vi "TTA_MATLAB_TX_Perform1RFIC1TxACPRTest.vi"(0 "Channel":string(combo), 1 "MXG VISA Resource In":refnum<visa-resource-name>, 2 "EXA VISA Resource":refnum<visa-resource-name>, 5 "Tx":string(combo), 7 "Active ACPR Refnum":refnum<vi>, 11 "error in":errorcluster) -> (4 "ACPR\nResults":T1, 12 "MXG VISA Resource Out":refnum<visa-resource-name>, 13 "EXA VISA Resource Out":refnum<visa-resource-name>, 15 "error out":errorcluster)   [LabVIEW 2016]
uses:
  TTA_Globals/TTA_Global_Complete_Settings.vi
panel:
  out "RFPAL PMU\nResults":dbl[](array[numeric])
  out "RF Frequency":dbl[](array[numeric])
  out "ACPR Data":dbl[][](array[numeric])
  out "In Range?":bool[](array[boolean])
  out "Amp Max\nSpec (dBm)":dbl
  out "Amp Min\nSpec (dBm)":dbl
  out "IF Index":i32
  in  "PALLinearization Values":T2
  out "Tx#":i32
  out "CH#":i32
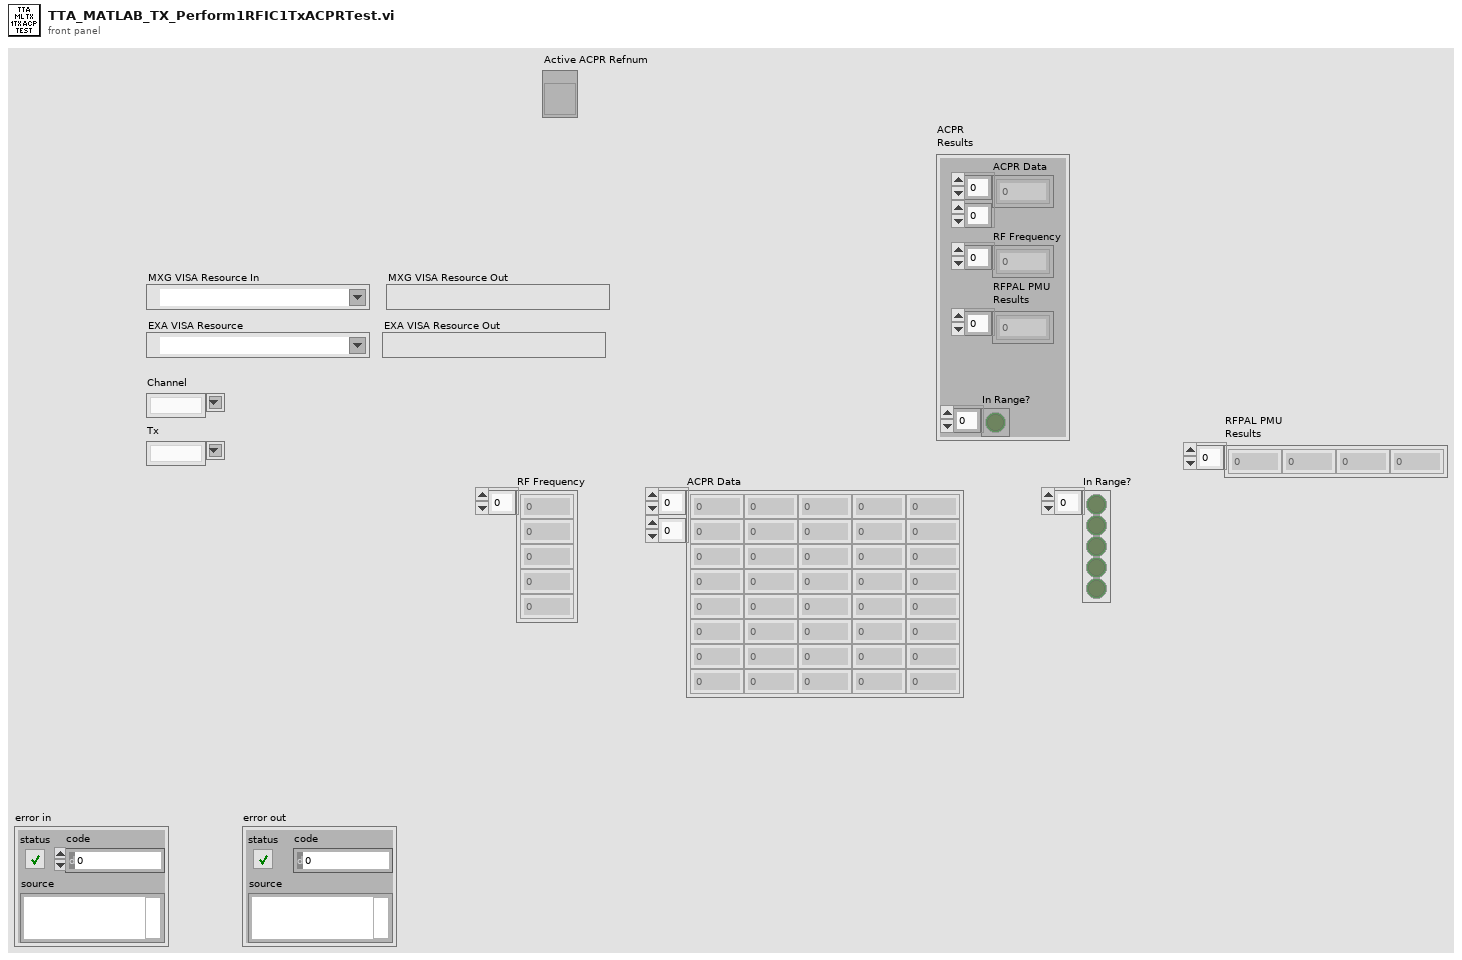
[diagram p1: front panel]
types:
  T1 = cluster{"ACPR Data":dbl[][], "RF Frequency":dbl[], "RFPAL PMU\nResults":dbl[], "In Range?":bool[]}
  T2 = cluster{"Tx IF Offsets":dbl[], "ACPR Filename":string, "Sampling Rate":dbl, "TxIF_Freq":dbl, "Power (dBm)":dbl, "IF Frequency Sweep (MHz)":dbl[], "BDSFreq":dbl, "Amplitude Range\nMax(dBm)":dbl, "Amplitude Range\nMin(dBm)":dbl, "CAL Amplitude\nIncrement(dB)":dbl, "CAL Amplitude\nDecrement (dB)":dbl, "Amplitude Least\nCriteria (dBm)":dbl}
  T3 = typedef "TTA_Control_Complete_Settings_Cluster.ctl" = cluster{"Brief Cluster":cluster{"STM Firmware File":string, "STM Firmware Address":string, "Required SW Version":string, "Template Used":string}, "Instrument Setting Cluster":cluster{"BDSFreq":dbl, "BDS Amp":dbl, "TxRFCal_Freq":dbl, "TxRFCal_Amp":dbl, "RxRFCal_Freq":dbl, "RxRFCal_Freq":dbl, "TxIF_Freq":dbl, "TxIF_Amp":dbl, "Tx_Output_Power_Signal_Freq":dbl, "Tx_ACPR_Signal_Freq":dbl, "Rx_RF_Freq":dbl, "Rx_RF_Amp":dbl, "Rx_Output_Power_Signal_Freq":dbl, "Rx_Output_Power_Sense_Freq":dbl}, "PAL Calibration\nInputs Cluster":cluster{"Amplitude Range\nMax(dBm)":dbl, "Amplitude Range\nMin(dBm)":dbl, "Amplitude Least\nCriteria (dBm)":dbl, "Frequency 1":dbl, "Frequency 2":dbl, "Frequency 3":dbl, "CAL Amplitude\nDecrement (dB)":dbl, "CAL Amplitude\nIncrement(dB)":dbl, "DownloadFile":string}, "TxOffset Cal Cluster":cluster{"Tx1 Offset (dB)":dbl, "Tx2 Offset (dB)":dbl, "Tx3 Offset (dB)":dbl, "Tx4 Offset (dB)":dbl, "Total RF Tx Loss (dB)":dbl}, "RxOffset Cal Cluster":cluster{"Rx1 Offset (dB)":dbl, "Rx2 Offset (dB)":dbl, "Rx3 Offset (dB)":dbl, "Rx4 Offset (dB)":dbl, "Total RF Rx Loss (dB)":dbl}, "TX Output Power Settings Cluster":cluster{"Frequency Sweep (MHz)":dbl[], "Sig Gen \nPower (dBm)":dbl, "Span (kHz)":dbl, "RBW (Hz)":dbl, "Ref Level (dBm)":dbl, "Low Power \nLimit":dbl, "High Power \nLimit":dbl, "DigAtt Max":dbl, "DigAtt Min":dbl}, "Tx ACPR Settings Cluster":cluster{"ACPR Filename":string, "Sampling Rate":dbl, "Power (dBm)":dbl, "IF Frequency Sweep (MHz)":dbl[], "State Name":string, "Mechanical\nAttenuation":dbl, "RefLevel Offset":dbl, "Amplitude Range\nMax (dBm)":dbl, "Amplitude Range\nMin (dBm)":dbl, "Cal Amp \nIncrement (dB)":dbl, "Cal Amp\nDecrement (dB)":dbl}, "Power Cal Cluster":cluster{"Power List (dBm)":dbl[], "Frequency (MHz)":dbl[], "Cal Decrement (dB)":dbl, "Cal Increment (dB)":dbl}, "Rx Received Power Settings Cluster":cluster{"Frequency Sweep (MHz)":dbl[], "Power (dBm)":dbl, "Span (kHz)":dbl, "RBW (Hz)":dbl, "Ref Level":dbl, "Low Power \nLimit (dBm)":dbl, "High Power\nLimit (dBm)":dbl}, "Tx Output Power Criteria Cluster":cluster{"CH1-TX1 \nMin":dbl, "CH1-TX1\nMax":dbl, "CH1-TXx3\nMin ":dbl, "CH1-TXx3\nMax":dbl, "CH2-TX1\nMin":dbl, "CH2-TX1\nMax":dbl, "CH2-TXx3\nMin":dbl, "CH2-TXx3\nMax":dbl}, "Tx ACPR Criteria Cluster":cluster{"Min Inband":dbl, "Max Close Outband":dbl, "Max Far Outband":dbl}, "Rx Output Power Criteria Cluster":cluster{"CH1-RX1 \nMin":dbl, "CH1-RX1 \nMax":dbl, "CH1-RXx3 \nMin":dbl, "CH1-RXx3\nMax":dbl, "CH2-RX1\nMin":dbl, "CH2-RX1\nMax":dbl, "CH2-RXx3\nMin":dbl, "CH2-RXx3\nMax":dbl}}
  T4 = cluster{"BDSFreq":dbl, "BDS Amp":dbl, "TxRFCal_Freq":dbl, "TxRFCal_Amp":dbl, "RxRFCal_Freq":dbl, "RxRFCal_Freq":dbl, "TxIF_Freq":dbl, "TxIF_Amp":dbl, "Tx_Output_Power_Signal_Freq":dbl, "Tx_ACPR_Signal_Freq":dbl, "Rx_RF_Freq":dbl, "Rx_RF_Amp":dbl, "Rx_Output_Power_Signal_Freq":dbl, "Rx_Output_Power_Sense_Freq":dbl}
  T5 = cluster{"Amplitude Range\nMax(dBm)":dbl, "Amplitude Range\nMin(dBm)":dbl, "Amplitude Least\nCriteria (dBm)":dbl, "Frequency 1":dbl, "Frequency 2":dbl, "Frequency 3":dbl, "CAL Amplitude\nDecrement (dB)":dbl, "CAL Amplitude\nIncrement(dB)":dbl, "DownloadFile":string}
  T6 = cluster{"Tx1 Offset (dB)":dbl, "Tx2 Offset (dB)":dbl, "Tx3 Offset (dB)":dbl, "Tx4 Offset (dB)":dbl, "Total RF Tx Loss (dB)":dbl}
  T7 = cluster{"ACPR Filename":string, "Sampling Rate":dbl, "Power (dBm)":dbl, "IF Frequency Sweep (MHz)":dbl[], "State Name":string, "Mechanical\nAttenuation":dbl, "RefLevel Offset":dbl, "Amplitude Range\nMax (dBm)":dbl, "Amplitude Range\nMin (dBm)":dbl, "Cal Amp \nIncrement (dB)":dbl, "Cal Amp\nDecrement (dB)":dbl}
  T8 = cluster{"CH1-TX1 \nMin":dbl, "CH1-TX1\nMax":dbl, "CH1-TXx3\nMin ":dbl, "CH1-TXx3\nMax":dbl, "CH2-TX1\nMin":dbl, "CH2-TX1\nMax":dbl, "CH2-TXx3\nMin":dbl, "CH2-TXx3\nMax":dbl}
  T9 = cluster{"Min Inband":dbl, "Max Close Outband":dbl, "Max Far Outband":dbl}
  T10 = cluster{"Amplitude Range\nMax (dBm)":dbl, "Amplitude Range\nMin (dBm)":dbl, "Cal Amp\nDecrement (dB)":dbl, "Cal Amp \nIncrement (dB)":dbl, "Amplitude Least\nCriteria (dBm)":dbl}
  T11 = enum16{"TX1", "TX2", "TX3", "TX4", "TXx3", "TXx4", "RX1", "RX2", "RX3", "RX4", "RXx3", "RXx4", "RFCal"}
  T12 = cluster{"RF Frequency":dbl, "RFPAL PMU\nResults":dbl[], "ACPR Data ":dbl[][]}
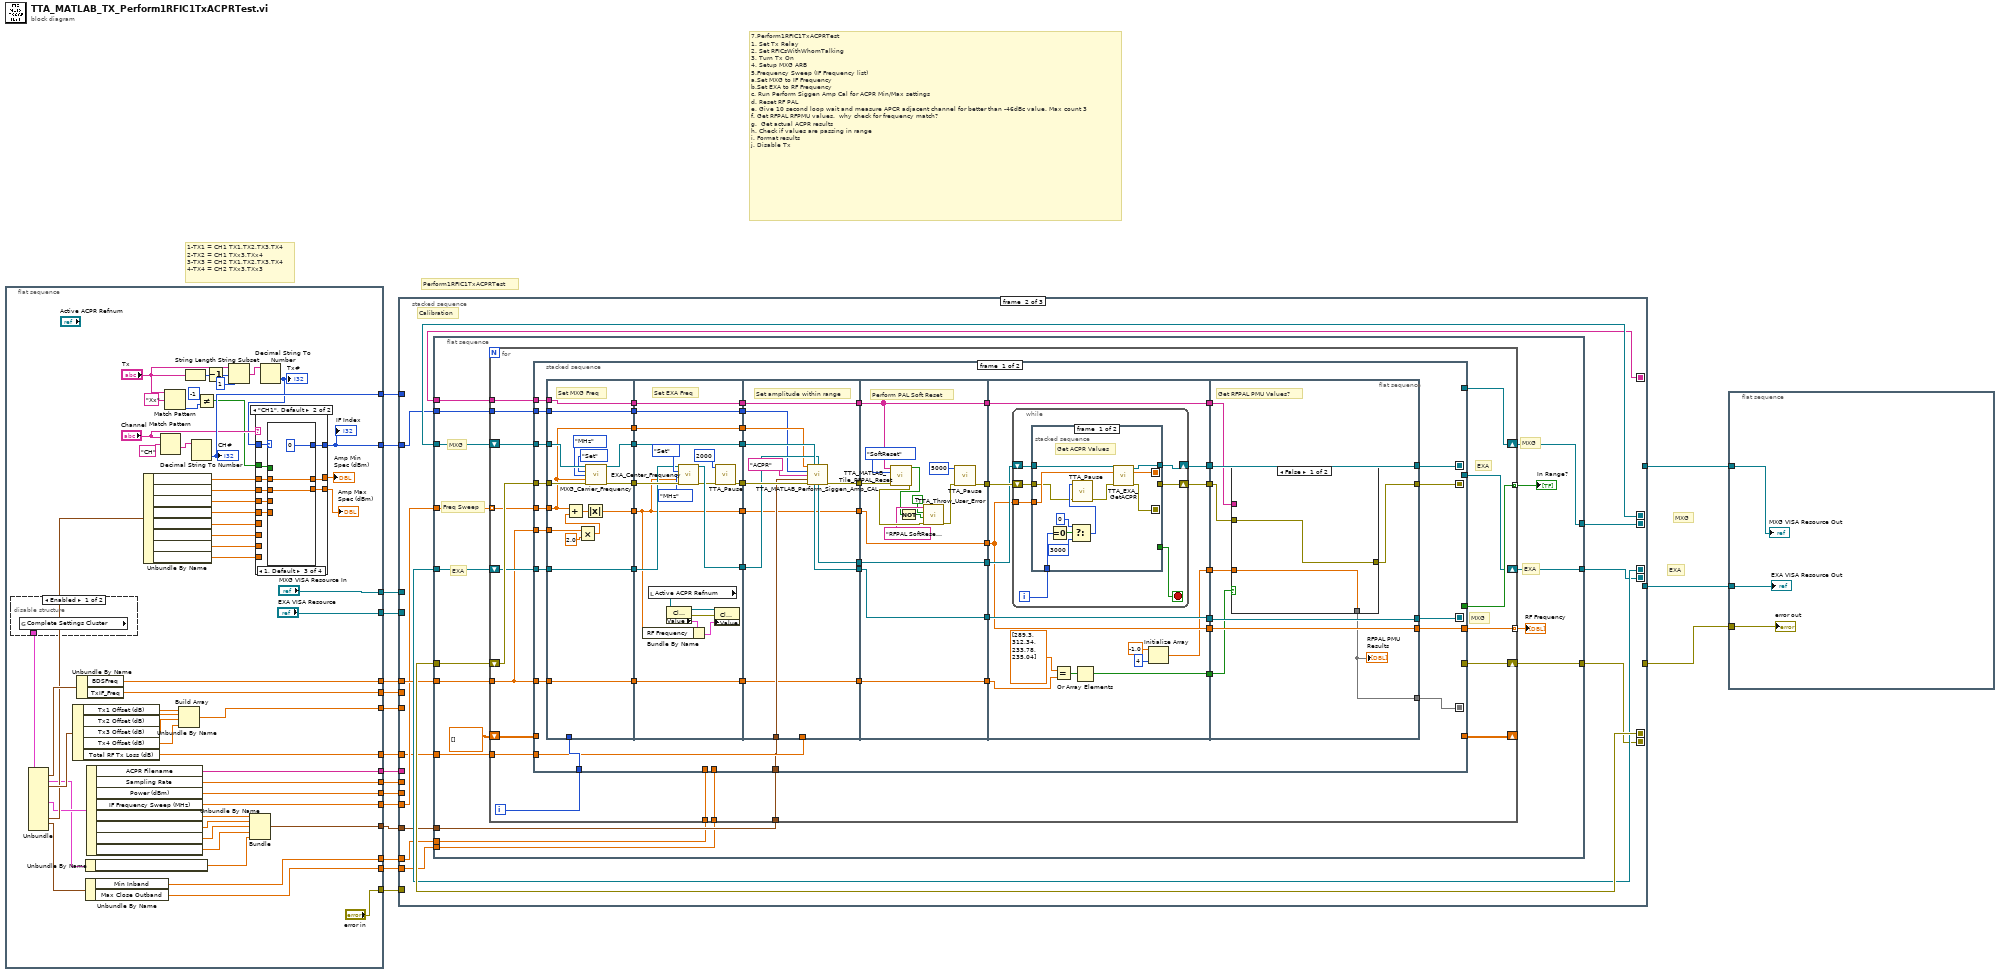
[diagram p0: block diagram]
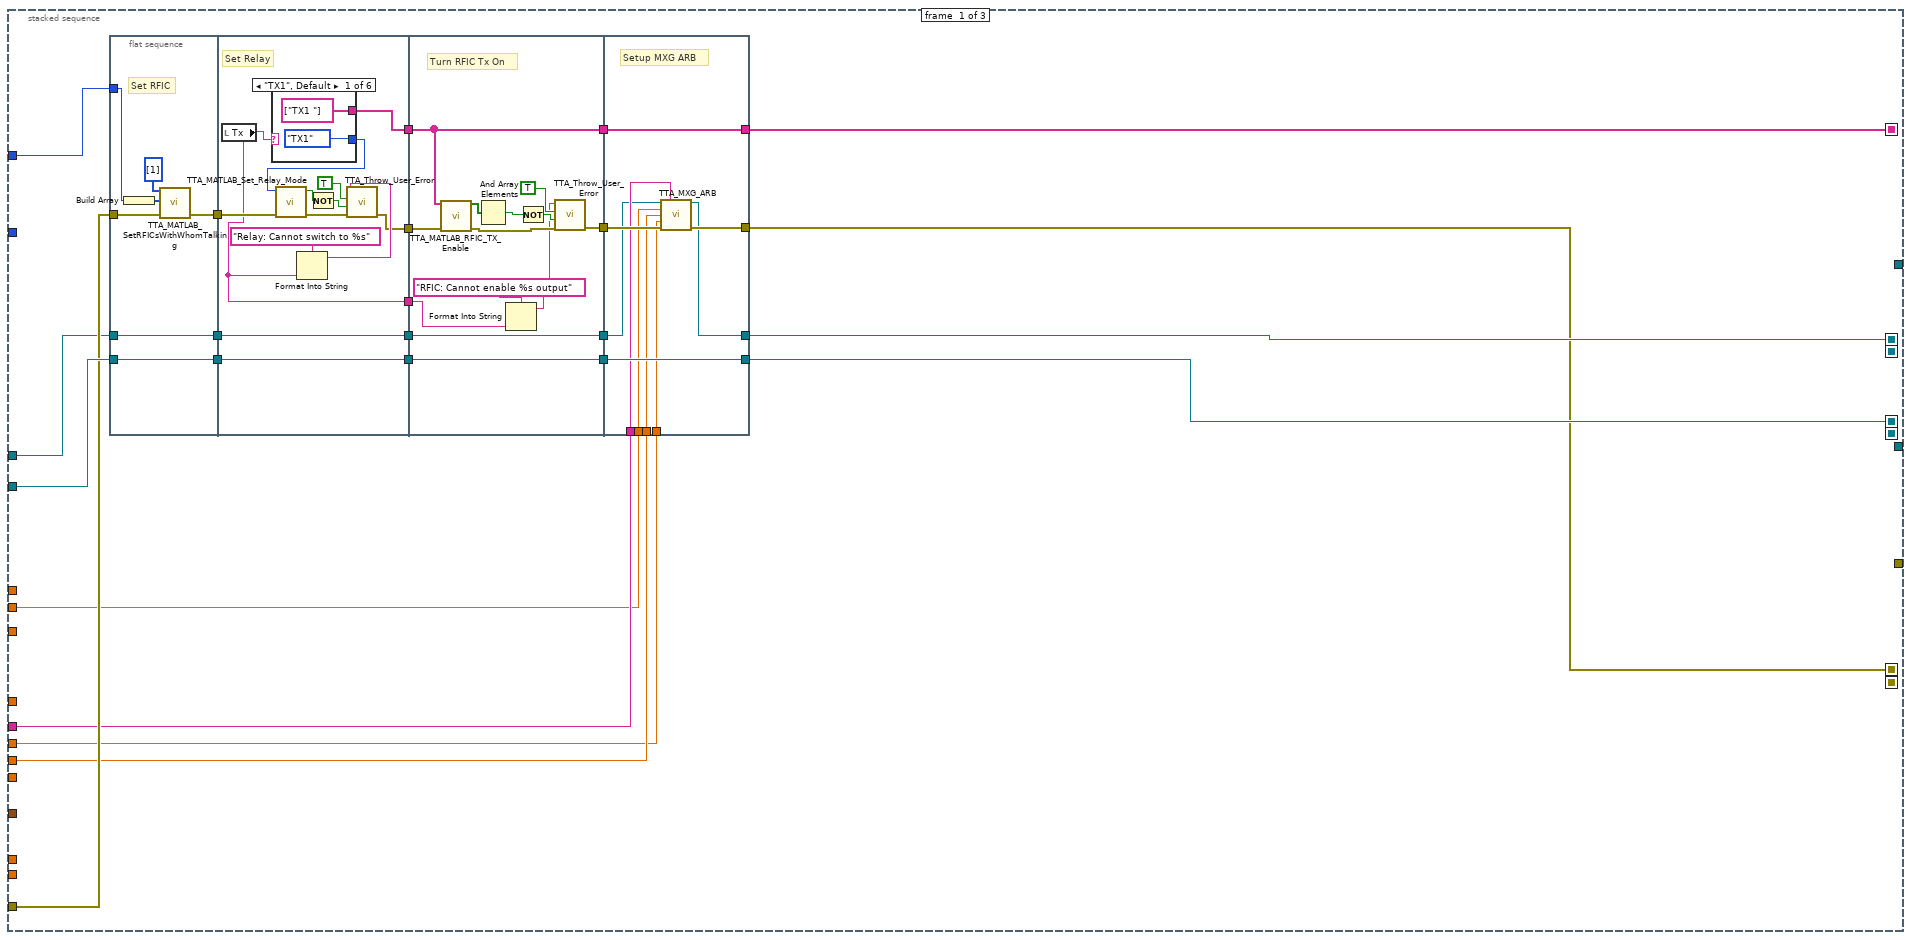
[diagram p2: hidden frame]
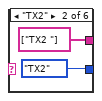
[diagram p3: hidden frame]
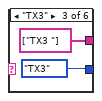
[diagram p4: hidden frame]
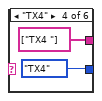
[diagram p5: hidden frame]
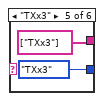
[diagram p6: hidden frame]
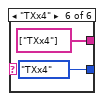
[diagram p7: hidden frame]
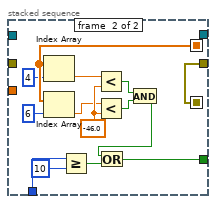
[diagram p8: hidden frame]
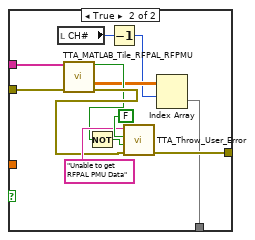
[diagram p9: hidden frame]
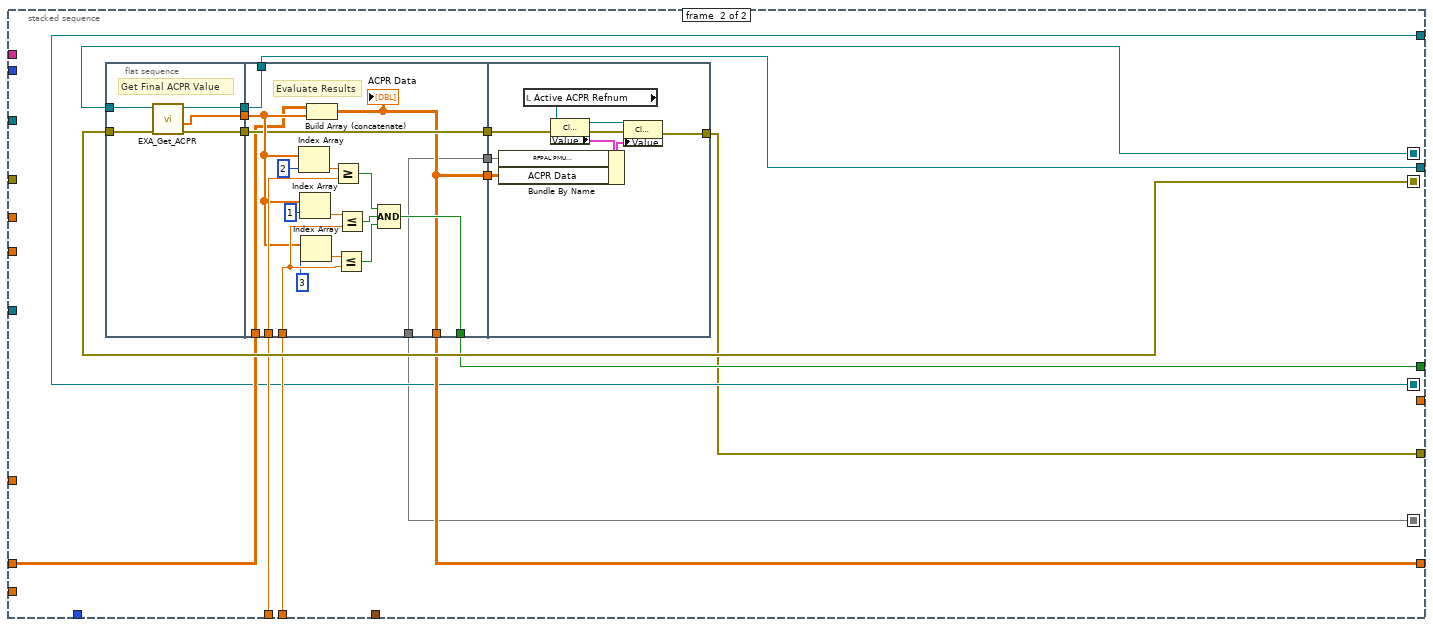
[diagram p10: hidden frame]
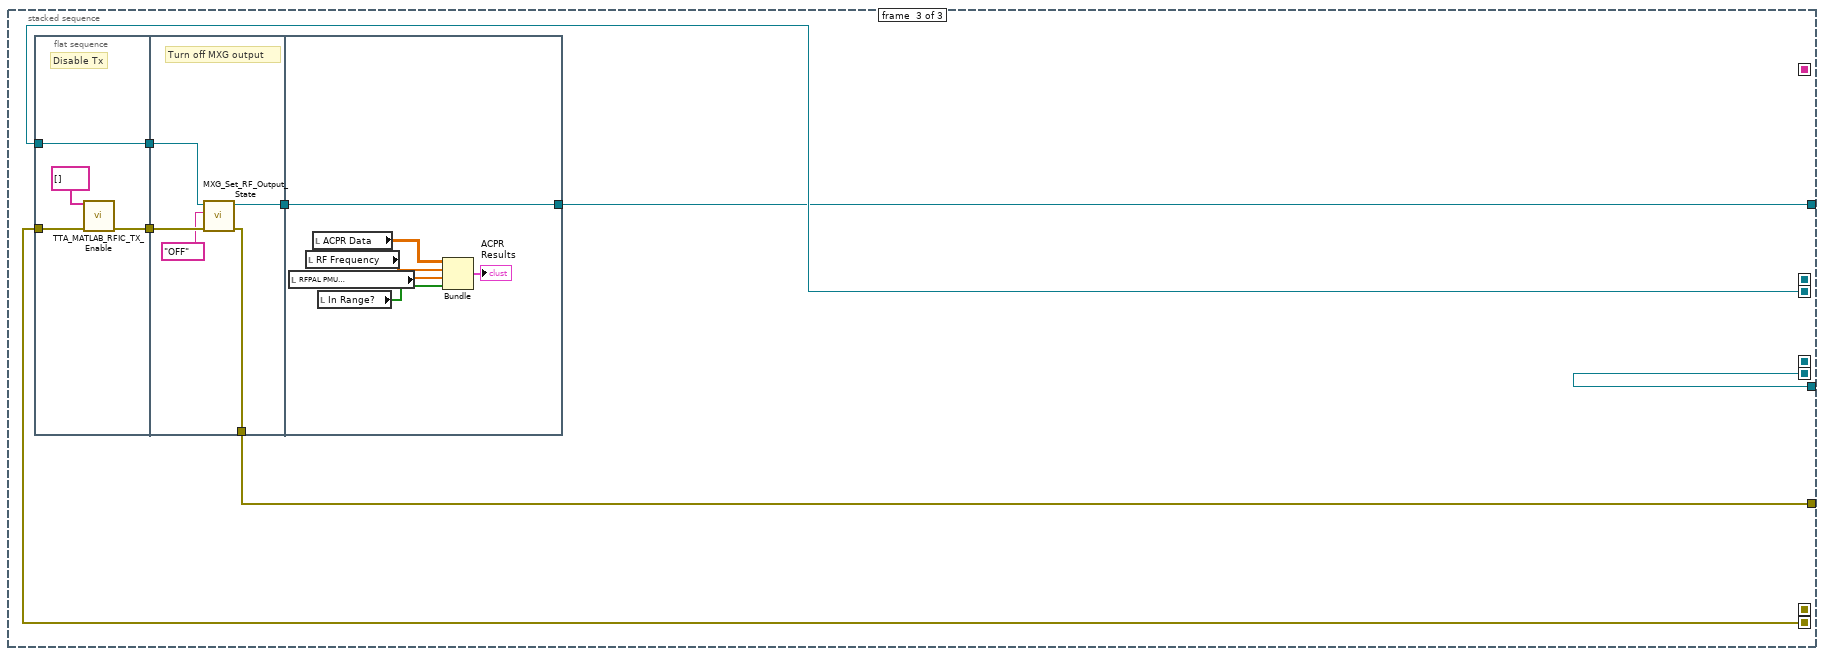
[diagram p11: hidden frame]
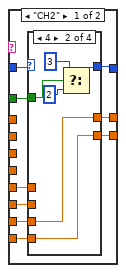
[diagram p12: hidden frame]
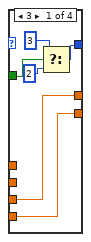
[diagram p13: hidden frame]
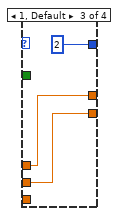
[diagram p14: hidden frame]
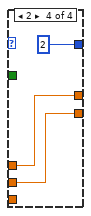
[diagram p15: hidden frame]
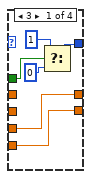
[diagram p16: hidden frame]
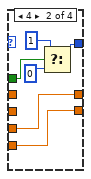
[diagram p17: hidden frame]
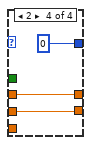
[diagram p18: hidden frame]
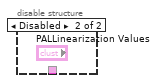
[diagram p19: hidden frame]
diagram:
  # "Perform1RFIC1TxACPRTest"
  # "7.Perform1RFIC1TxACPRTest\n1. Set Tx Relay\n2. Set RFICsWithWhomTalking\n3. Turn Tx On\n4. Setup MXG ARB\n5.Frequency Sweep (IF Frequency list)\na.Set MXG to IF Frequency\nb.Set EXA to RF Frequency\nc. Run Perform Siggen Amp Cal for ACPR Min/Max settings\nd. Reset RF PAL\ne. Give 10 second loop wait and measure APCR adjacent channel for better than -46dBc value. Max count 3\nf. Get RFPAL RFPMU values.  why check for frequency match?\ng.  Get actual ACPR results\nh. Check if values are passing in range\ni. Format results\nj. Disable Tx"
  # "1-TX1 = CH1 TX1,TX2,TX3,TX4\n2-TX2 = CH1 TXx3,TXx4\n3-TX3 = CH2 TX1,TX2,TX3,TX4\n4-TX4 = CH2 TXx3,TXx3"
  # "EXA"
  # "MXG"
  n1 = flat-sequence {
    tunnel: ["error in"] -> w19
    tunnel: ["MXG VISA Resource In"] -> w17
    tunnel: ["EXA VISA Resource"] -> w16
    tunnel: [w69] -> w18
    tunnel: [w55] -> w13
    tunnel: [w56] -> w12
    tunnel: [w61] -> w11
    tunnel: [w47] -> w10
    tunnel: [w33] -> w9
    tunnel: [w46] -> w8
    tunnel: [w32] -> w6
    tunnel: [w31] -> w5
    tunnel: [w30] -> w4
    tunnel: [w23] -> w3
    tunnel: [w21] -> w2
    tunnel: [w20] -> w1
    frame #0 {
      n2 = disable-structure shown="Enabled" {
        disable-tunnel: [w129 _] -> w64
        frame Enabled {
          n3 = global read "TTA_Global_Complete_Settings.vi" "Complete Settings Cluster"() -> (w129:T3)
        }
        frame Disabled {
        }
      }
      n4 = Unbundle(w64) -> ("Instrument Setting Cluster"=w63:T4, "PAL Calibration\nInputs Cluster"=w29:T5, "TxOffset Cal Cluster"=w62:T6, "Tx ACPR Settings Cluster"=w34:T7, "Tx Output Power Criteria Cluster"=w45:T8, "Tx ACPR Criteria Cluster"=w22:T9)  [unwired: 6 out]
      n5 = Unbundle By Name(w62) -> ("Tx1 Offset (dB)"=w60:dbl, "Tx2 Offset (dB)"=w59:dbl, "Tx3 Offset (dB)"=w58:dbl, "Tx4 Offset (dB)"=w57:dbl, "Total RF Tx Loss (dB)"=w46:dbl)
      n6 = Unbundle By Name(w63) -> ("BDSFreq"=w61:dbl, "TxIF_Freq"=w55:dbl)
      n7 = Unbundle By Name(w29) -> ("Amplitude Least\nCriteria (dBm)"=w24:dbl)
      n8 = Unbundle By Name(w22) -> ("Min Inband"=w21:dbl, "Max Close Outband"=w20:dbl)
      n9 = Unbundle By Name(w34) -> ("ACPR Filename"=w32:string, "Sampling Rate"=w30:dbl, "Power (dBm)"=w31:dbl, "IF Frequency Sweep (MHz)"=w33:dbl[], "Amplitude Range\nMax (dBm)"=w28:dbl, "Amplitude Range\nMin (dBm)"=w27:dbl, "Cal Amp\nDecrement (dB)"=w26:dbl, "Cal Amp \nIncrement (dB)"=w25:dbl)
      n10 = Unbundle By Name(w45) -> ("CH1-TX1 \nMin"=w44:dbl, "CH1-TX1\nMax"=w43:dbl, "CH1-TXx3\nMin"=w42:dbl, "CH1-TXx3\nMax"=w41:dbl, "CH2-TX1\nMin"=w40:dbl, "CH2-TX1\nMax"=w39:dbl, "CH2-TXx3\nMin"=w38:dbl, "CH2-TXx3\nMax"=w37:dbl)
      n11 = Match Pattern(string="Channel", regular expression="CH") -> (after substring=w70:string)  [unwired: 1 in, 3 out]
      n12 = Match Pattern(string="Tx", regular expression="Xx") -> (offset past match=w50:i32)  [unwired: 1 in, 3 out]
      n13 = Build Array(w60, w59, w58, w57) -> (w56:dbl[])
      n14 = String Length(string="Tx") -> (length=w68:i32)
      n15 = Decimal String To Number(string=w70) -> (number=w69:i32)  [unwired: 2 in, 1 out]
      "CH#" <- w69
      n16 = Not Equal?(x=-1, y=w50) -> (x != y?=w48:bool)
      n17 = Decrement(x=w68) -> (x-1=w67:i32)
      n18 = String Subset(string="Tx", offset (0)=w67, length (rest)=1 ("length (rest)")) -> (substring=w65:string)
      n19 = Bundle("Amplitude Range\nMax (dBm)"=w28, "Amplitude Range\nMin (dBm)"=w27, "Cal Amp\nDecrement (dB)"=w26, "Cal Amp \nIncrement (dB)"=w25, "Amplitude Least\nCriteria (dBm)"=w24) -> (w23:T10)  [unwired: 1 in]
      n20 = Decimal String To Number(string=w65) -> (number=w53:i32)  [unwired: 2 in, 1 out]
      "Tx#" <- w53
      n21 = case shown="\"CH1\", Default" "Channel" {
        tunnel: w53 -> [w82 w110]
        tunnel: [w83 w109] -> w47
        tunnel: w48 -> [w81 w108]
        tunnel: w44 -> [_ w107]
        tunnel: w43 -> [_ w106]
        tunnel: w42 -> [_ w105]
        tunnel: w41 -> [_ w104]
        tunnel: w40 -> [w80 _]
        tunnel: w39 -> [w79 _]
        tunnel: w38 -> [w78 _]
        tunnel: w37 -> [w77 _]
        tunnel: [w76 w103] -> w36
        tunnel: [w75 w102] -> w35
        frame "CH2" {
          n22 = case shown="4" w82 {
            tunnel: [w87 w93 2 2] -> w83
            tunnel: w81 -> [w86 w92 _ _]
            tunnel: w80 -> [_ _ w97 w100]
            tunnel: [w85 w91 w97 w100] -> w76
            tunnel: w79 -> [_ _ w96 w99]
            tunnel: [w84 w90 w96 w99] -> w75
            tunnel: w78 -> [w85 w91 _ _]
            tunnel: w77 -> [w84 w90 _ _]
            frame 3 {
              n23 = Select(t=3, s=w86, f=2) -> (s? t:f=w87:i32)
            }
            frame 4 {
              n24 = Select(t=3, s=w92, f=2) -> (s? t:f=w93:i32)
            }
            frame 1, Default {
            }
            frame 2 {
            }
          }
        }
        frame "CH1", Default {
          n25 = case shown="1, Default" w110 {
            tunnel: [w114 w120 0 0] -> w109
            tunnel: w108 -> [w113 w119 _ _]
            tunnel: [w112 w118 w124 w127] -> w103
            tunnel: w107 -> [_ _ w124 w127]
            tunnel: [w111 w117 w123 w126] -> w102
            tunnel: w106 -> [_ _ w123 w126]
            tunnel: w105 -> [w112 w118 _ _]
            tunnel: w104 -> [w111 w117 _ _]
            frame 3 {
              n26 = Select(t=1, s=w113, f=0) -> (s? t:f=w114:i32)
            }
            frame 4 {
              n27 = Select(t=1, s=w119, f=0) -> (s? t:f=w120:i32)
            }
            frame 1, Default {
            }
            frame 2 {
            }
          }
        }
      }
      "IF Index" <- w47
      "Amp Min\nSpec (dBm)" <- w36
      "Amp Max\nSpec (dBm)" <- w35
    }
  }
  n28 = stacked-sequence {
    seq-local: [w130 _ _] -> [_ w222 _]
    seq-local: [w142 _ _] -> [_ w219 _]
    seq-local: [w143 _ _] -> [_ w221 _]
    seq-local: [_ w216 _] -> [_ _ w492]
    seq-local: [_ w214 _] -> [_ _ w498]
    seq-local: [_ w215 _] -> [_ _ w495]
    seq-local: [w131 _ _] -> [_ w211 _]
    tunnel: w19 -> [w141 _ _]
    tunnel: w18 -> [w153 _ _]
    tunnel: w17 -> [w140 _ _]
    tunnel: w16 -> [w151 _ _]
    tunnel: [_ _ w495] -> w15
    tunnel: [_ _ w494] -> w14
    tunnel: w13 -> [w134 _ _]
    tunnel: w12 -> [_ _ _]
    tunnel: w11 -> [_ w220 _]
    tunnel: w10 -> [_ w213 _]
    tunnel: w9 -> [_ w218 _]
    tunnel: w8 -> [_ w217 _]
    tunnel: [_ _ w496] -> w7
    tunnel: w6 -> [w135 _ _]
    tunnel: w5 -> [w133 _ _]
    tunnel: w4 -> [w132 _ _]
    tunnel: w3 -> [_ w212 _]
    tunnel: w2 -> [_ w210 _]
    tunnel: w1 -> [_ w209 _]
    frame #0 {
      n29 = flat-sequence {
        tunnel: [w157] -> w152
        tunnel: [w154] -> w150
        tunnel: [w156] -> w149
        tunnel: w153 -> [w158]
        tunnel: w151 -> [w156]
        tunnel: w141 -> [w155]
        tunnel: w140 -> [w154]
        tunnel: w152 -> [w173]
        tunnel: w150 -> [w165]
        tunnel: w149 -> [w163]
        tunnel: [w165] -> w148
        tunnel: [w161] -> w147
        tunnel: [w164] -> w146
        tunnel: [w163] -> w145
        tunnel: [w162] -> w144
        tunnel: w148 -> [w187]
        tunnel: w147 -> [w191]
        tunnel: w146 -> [w190]
        tunnel: w145 -> [w189]
        tunnel: w144 -> [w188]
        tunnel: [w189] -> w139
        tunnel: [w191] -> w138
        tunnel: [w187] -> w137
        tunnel: [w186] -> w136
        tunnel: [w199] -> w142
        tunnel: [w207] -> w131
        tunnel: [w208] -> w143
        tunnel: w139 -> [w208]
        tunnel: w138 -> [w207]
        tunnel: w137 -> [w204]
        tunnel: w136 -> [w206]
        tunnel: w135 -> [w205]
        tunnel: w134 -> [w203]
        tunnel: w133 -> [w202]
        tunnel: w132 -> [w201]
        tunnel: [w200] -> w130
        frame #0 {
          # "Set RFIC"
          n30 = Build Array(w158) -> (w159:i32[])
          n31 = call "TTA_MATLAB_SetRFICsWithWhomTalking.vi"("Panel Array"=i32[] [1], "RFIC Array"=w159, "error in"=w155) -> ("error out"=w157:errorcluster)  [unwired: 12 in]
        }
        frame #1 {
          # "Set Relay"
          n32 = local read "Tx"() -> (w162:string)
          n33 = case shown="\"TX1\", Default" w162 {
            tunnel: [T11."TX1" ("Mode") T11."TX2" ("Mode") T11."TX3" ("Mode") T11."TX4" ("Mode") T11."TXx3" ("Mode") T11."TXx4" ("Mode")] -> w172
            tunnel: [string[] ["TX1 "] ("Channels") string[] ["TX2 "] ("Channels") string[] ["TX3 "] ("Channels") string[] ["TX4 "] ("Channels") string[] ["TXx3"] ("Channels") string[] ["TXx4"] ("Channels")] -> w161
            frame "TX1", Default {
            }
            frame "TX2" {
            }
            frame "TX3" {
            }
            frame "TX4" {
            }
            frame "TXx3" {
            }
            frame "TXx4" {
            }
          }
          n34 = call "TTA_MATLAB_Set_Relay_Mode.vi"("error in"=w173, "Mode"=w172) -> ("error out"=w171:errorcluster, "Success"=w170:bool)  [unwired: 8 in]
          n35 = Format Into String(format string="Relay: Cannot switch to %s", w162) -> (resulting string=w166:string)  [unwired: 2 in, 1 out]
          n36 = Not(x=w170) -> (.not. x?=w169:bool)
          n37 = call "TTA_Throw_User_Error.vi"("error in"=w171, "Error?"=w169, "Stop Execution on Fail"=TRUE, "Error Message"=w166) -> ("error out"=w164:errorcluster)  [unwired: 7 in]
        }
        frame #2 {
          # "Turn RFIC Tx On"
          n38 = call "TTA_MATLAB_RFIC_TX_Enable.vi"("Channels"=w191, "error in"=w190) -> ("SuccessComm"=w198:bool[], "error out"=w194:errorcluster)  [unwired: 12 in]
          n39 = And Array Elements(Boolean array=w198) -> (logical AND=w195:bool)
          n40 = Format Into String(format string="RFIC: Cannot enable %s output", w188) -> (resulting string=w192:string)  [unwired: 2 in, 1 out]
          n41 = Not(x=w195) -> (.not. x?=w196:bool)
          n42 = call "TTA_Throw_User_Error.vi"("error in"=w194, "Error?"=w196, "Stop Execution on Fail"=TRUE, "Error Message"=w192) -> ("error out"=w186:errorcluster)  [unwired: 7 in]
        }
        frame #3 {
          # "Setup MXG ARB"
          n43 = call "TTA_MXG_ARB.vi"("VISA resource In"=w204, "Waveform File"=w205, "Frequency (MHz)"=w203, "Output Power\nLevel (dBm)"=w202, "ARB Sample Rate"=w201, "error in"=w206) -> ("VISA resource Out"=w199:refnum<visa-resource-name>, "error out"=w200:errorcluster)  [unwired: 8 in]
        }
      }
    }
    frame #1 {
      # "Calibration"
      n44 = flat-sequence {
        tunnel: w222 -> [w239]
        tunnel: w221 -> [w238]
        tunnel: [w237] -> w215
        tunnel: [w236] -> w216
        tunnel: w220 -> [w235]
        tunnel: w218 -> [w234]
        tunnel: w219 -> [w233]
        tunnel: w217 -> [w232]
        tunnel: [w231] -> w214
        tunnel: w213 -> [w229]
        tunnel: w212 -> [w228]
        tunnel: w211 -> [w227]
        tunnel: w210 -> [w226]
        tunnel: w209 -> [w225]
        frame #0 {
          # "EXA"
          # "MXG"
          # "Freq Sweep"
          # "EXA"
          # "MXG"
          n45 = for {
            shift-right: [w241] -> w236
            shift-left: w239 -> [w256]
            shift-right: [w244] -> w237
            shift-left: w238 -> [w255]
            tunnel: w235 -> [w240]
            tunnel: w234 -> [w254] mode=indexing
            shift-right: [w242] -> w231
            shift-left: w233 -> [w257]
            tunnel: w232 -> [w253]
            tunnel: [w246] -> w230 mode=indexing
            tunnel: w229 -> [w252]
            tunnel: w228 -> [w251]
            tunnel: w227 -> [w250]
            tunnel: w226 -> [w249]
            tunnel: w225 -> [w248]
            shift-right: [w247] -> _
            shift-left: dbl[][] [] -> [w243]
            tunnel: [w245] -> w224 mode=indexing
            i -> [w258]
            # "EXA"
            # "MXG"
            n46 = stacked-sequence {
              seq-local: [w276 _] -> [_ w458]
              seq-local: [w273 _] -> [_ w448]
              seq-local: [w271 _] -> [_ w459]
              seq-local: [w266 _] -> [_ w444]
              tunnel: w258 -> [w287 _]
              tunnel: w240 -> [w286 _]
              tunnel: w257 -> [w285 _]
              tunnel: w256 -> [w284 _]
              tunnel: w255 -> [w283 _]
              tunnel: w254 -> [w282 _]
              tunnel: w253 -> [w281 _]
              tunnel: w252 -> [w280 _]
              tunnel: w251 -> [w279 _]
              tunnel: w250 -> [w278 _]
              tunnel: w249 -> [_ w454]
              tunnel: w248 -> [_ w453]
              tunnel: [_ w452] -> w247
              tunnel: [_ w451] -> w246
              tunnel: [w267 _] -> w245
              tunnel: [_ w450] -> w244
              tunnel: w243 -> [_ w449]
              tunnel: [_ w448] -> w242
              tunnel: [_ w446] -> w241
              tunnel: w240 -> [w264 _]
              frame #0 {
                n47 = flat-sequence {
                  tunnel: w282 -> [w313]
                  tunnel: w287 -> [_]
                  tunnel: w286 -> [w321]
                  tunnel: w285 -> [w324]
                  tunnel: w284 -> [w325]
                  tunnel: w283 -> [w315]
                  tunnel: [w317] -> w309
                  tunnel: [w316] -> w308
                  tunnel: [w315] -> w307
                  tunnel: [w314] -> w306
                  tunnel: [w313] -> w305
                  tunnel: w280 -> [w312]
                  tunnel: [w312] -> w304
                  tunnel: w278 -> [w311]
                  tunnel: [w311] -> w303
                  tunnel: [w310] -> w265
                  tunnel: w264 -> [w310]
                  tunnel: w309 -> [w327]
                  tunnel: w308 -> [w344]
                  tunnel: w307 -> [w342]
                  tunnel: w306 -> [w339]
                  tunnel: [w340] -> w302
                  tunnel: [w339] -> w301
                  tunnel: [w336] -> w300
                  tunnel: [w335] -> w299
                  tunnel: w305 -> [w335]
                  tunnel: [w334] -> w298
                  tunnel: w304 -> [w334]
                  tunnel: [w333] -> w297
                  tunnel: w303 -> [w333]
                  tunnel: [w327] -> w296
                  tunnel: w265 -> [w326]
                  tunnel: [w326] -> w261
                  tunnel: w302 -> [w354]
                  tunnel: w301 -> [w355]
                  tunnel: w300 -> [w357]
                  tunnel: w281 -> [_]
                  tunnel: w299 -> [w353]
                  tunnel: w298 -> [w352]
                  tunnel: w279 -> [w351]
                  tunnel: [w350] -> w295
                  tunnel: [w349] -> w294
                  tunnel: w297 -> [w349]
                  tunnel: [w348] -> w293
                  tunnel: [w347] -> w292
                  tunnel: w296 -> [w346]
                  tunnel: [w346] -> w291
                  tunnel: [w345] -> w262
                  tunnel: w261 -> [w345]
                  tunnel: w295 -> [w366]
                  tunnel: w294 -> [w359]
                  tunnel: w293 -> [w360]
                  tunnel: w292 -> [w361]
                  tunnel: [w364] -> w290
                  tunnel: w291 -> [w362]
                  tunnel: [w362] -> w289
                  tunnel: [w361] -> w288
                  tunnel: [w360] -> w275
                  tunnel: [w359] -> w269
                  tunnel: [w358] -> w263
                  tunnel: w262 -> [w358]
                  tunnel: w290 -> [w386]
                  tunnel: w289 -> [w380]
                  tunnel: w288 -> [w385]
                  tunnel: [w384] -> w277
                  tunnel: w275 -> [w383]
                  tunnel: [w383] -> w274
                  tunnel: [w382] -> w272
                  tunnel: [w381] -> w270
                  tunnel: w269 -> [w381]
                  tunnel: [w380] -> w268
                  tunnel: w263 -> [w379]
                  tunnel: [w376] -> w260
                  tunnel: [w373] -> w259
                  tunnel: w277 -> [w428]
                  tunnel: [w428] -> w276
                  tunnel: w274 -> [w427]
                  tunnel: [w427] -> w273
                  tunnel: w272 -> [w426]
                  tunnel: [w424] -> w271
                  tunnel: w270 -> [w425]
                  tunnel: [w420] -> w266
                  tunnel: w268 -> [w423]
                  tunnel: [w423] -> w267
                  tunnel: w260 -> [w422]
                  tunnel: w259 -> [w421]
                  frame #0 {
                    # "Set MXG Freq"
                    n48 = Multiply(x=w321, y=2.0) -> (x*y=w319:dbl)
                    n49 = Add(x=w313, y=w319) -> (x+y=w318:dbl)
                    n50 = Absolute Value(x=w318) -> (abs(x)=w317:dbl)
                    n51 = call "MXG_Carrier_Frequency.vi"("VISA resource name"=w324, "Mode"=enum16{"Set", "Get"}."Set", "Units"=enum16{"Hz", "kHz", "MHz", "GHz"}."MHz", "Frequency"=w313, "error in"=w325) -> ("VISA resource name"=w314:refnum<visa-resource-name>, "error out"=w316:errorcluster)  [unwired: 8 in, 1 out]
                  }
                  frame #1 {
                    # "Set EXA Freq"
                    n52 = local read "Active ACPR Refnum"() -> (w328:refnum<vi>)
                    n53 = property class="Clust (strict)"(reference=w328) -> (reference out=w331:refnum<vi>, error out=w330:errorcluster, "Value"=w329:T12)  [unwired: 1 in]
                    n54 = Bundle By Name(cluster=w329, "RF Frequency"=w327) -> (w332:T12)
                    n55 = call "EXA_Center_Frequency.vi"("VISA resource name"=w342, "Mode"=enum16{"Set", "Get"}."Set", "Units"=enum16{"Hz", "kHz", "MHz", "GHz"}."MHz", "Frequency"=w327, "error in"=w344) -> ("VISA resource name"=w340:refnum<visa-resource-name>, "error out"=w338:errorcluster)  [unwired: 8 in, 1 out]
                    n56 = property class="Clust (strict)"(reference=w331, error in=w330, "Value"=w332) -> ()  [unwired: 2 out]
                    n57 = call "TTA_Pause.vi"("error in"=w338, "Pause (ms)"=u32 2000) -> ("error out"=w336:errorcluster)  [unwired: 9 in]
                  }
                  frame #2 {
                    # "Set amplitude within range"
                    n58 = call "TTA_MATLAB_Perform_Siggen_Amp_CAL.vi"("IF Frequency (MHz)"=w353, "MXG VISA Resource In"=w355, "EXA VISA Resource"=w354, "IF Index"=w352, "Test"="ACPR", "Amp CAL Criteria Cluster"=w351, "error in"=w357) -> ("MXG VISA Resource Out"=w348:refnum<visa-resource-name>, "EXA VISA Resource Out"=w347:refnum<visa-resource-name>, "error out"=w350:errorcluster)  [unwired: 4 in, 2 out]
                  }
                  frame #3 {
                    # "Perform PAL Soft Reset"
                    n59 = call "TTA_MATLAB_Tile_RFPAL_Reset.vi"("Channels"=w359, "Mode"=enum16{"SoftReset", "HardReset"}."SoftReset", "error in"=w366) -> ("Success"=w370:bool, "error out"=w372:errorcluster)  [unwired: 9 in, 2 out]
                    n60 = Not(x=w370) -> (.not. x?=w369:bool)
                    n61 = call "TTA_Throw_User_Error.vi"("error in"=w372, "Error?"=w369, "Stop Execution on Fail"=TRUE, "Error Message"="RFPAL SoftReset not successful") -> ("error out"=w365:errorcluster)  [unwired: 7 in]
                    n62 = call "TTA_Pause.vi"("error in"=w365, "Pause (ms)"=u32 5000) -> ("error out"=w364:errorcluster)  [unwired: 9 in]
                  }
                  frame #4 {
                    n63 = while {
                      shift-right: [w387] -> w382
                      shift-left: w386 -> [w393]
                      tunnel: w380 -> [w392]
                      shift-right: [w389] -> w384
                      shift-left: w385 -> [w391]
                      i -> [w390]
                      stop <- w388 stop-if-true
                      n64 = stacked-sequence {
                        seq-local: [w402 _] -> [_ w416]
                        seq-local: [w395 _] -> [_ w406]
                        tunnel: w393 -> [w397 _]
                        tunnel: w392 -> [w405 _]
                        tunnel: w391 -> [w404 _]
                        tunnel: w390 -> [w401 w419]
                        tunnel: [w394 _] -> w389
                        tunnel: [_ w407] -> w388
                        tunnel: [_ w406] -> w387
                        frame #0 {
                          # "Get ACPR Values"
                          n65 = Equal To 0?(x=w401) -> (x = 0?=w400:bool)
                          n66 = Select(t=0, s=w400, f=3000) -> (s? t:f=w398:i32)
                          n67 = call "TTA_Pause.vi"("error in"=w397, "Pause (ms)"=w398) -> ("error out"=w403:errorcluster)  [unwired: 9 in]
                          n68 = call "TTA_EXA_GetACPR.vi"("VISA resource In"=w404, "Frequency (MHz)"=w405, "error in"=w403) -> ("VISA resource Out"=w394:refnum<visa-resource-name>, "ACP Values"=w402:dbl[], "error out"=w395:errorcluster)  [unwired: 9 in, 1 out]
                        }
                        frame #1 {
                          w413 = -46.0
                          n69 = Index Array(array=w416, index=4) -> (element=w412:dbl)
                          n70 = Index Array(array=w416, index=6) -> (element=w411:dbl)
                          n71 = Greater Or Equal?(x=w419, y=10) -> (x >= y?=w417:bool)
                          n72 = Less?(x=w412, y=w413) -> (x < y?=w409:bool)
                          n73 = Less?(x=w411, y=w413) -> (x < y?=w410:bool)
                          n74 = And(x=w409, y=w410) -> (x .and. y?=w408:bool)
                          n75 = Or(x=w408, y=w417) -> (x .or. y?=w407:bool)
                        }
                      }
                    }
                    n76 = Equal?(x=dbl[] [289.3, 312.34, 233.78, 235.04], y=w379) -> (x = y?=w377:bool[])
                    n77 = Or Array Elements(Boolean array=w377) -> (logical OR=w376:bool)
                    n78 = Initialize Array(-1.0 ("element"), 4 ("dimension size")) -> (w373:dbl[])
                  }
                  frame #5 {
                    # "Get RFPAL PMU Values?"
                    n79 = case shown="False" w422 {
                      tunnel: w426 -> [w430 w442]
                      tunnel: w425 -> [_ w441]
                      tunnel: [w430 w435] -> w424
                      tunnel: w421 -> [w429 _]
                      tunnel: [w429 w431] -> w420
                      frame False {
                      }
                      frame True {
                        n80 = local read "CH#"() -> (w433:i32)
                        n81 = call "TTA_MATLAB_Tile_RFPAL_RFPMU.vi"("Channels"=w441, "error in"=w442) -> ("Success"=w436:bool, "Tile Outputs"=w434:dbl[][], "error out"=w437:errorcluster)  [unwired: 9 in, 2 out]
                        n82 = Not(x=w436) -> (.not. x?=w439:bool)
                        n83 = Decrement(x=w433) -> (x-1=w432:i32)
                        n84 = call "TTA_Throw_User_Error.vi"("error in"=w437, "Error?"=w439, "Stop Execution on Fail"=FALSE, "Error Message"="Unable to get RFPAL PMU Data") -> ("error out"=w435:errorcluster)  [unwired: 7 in]
                        n85 = Index Array(array=w434, index (row)=w432) -> (element=w431:dbl[])  [unwired: 1 in]
                      }
                    }
                    "RFPAL PMU\nResults" <- w420
                  }
                }
              }
              frame #1 {
                n86 = flat-sequence {
                  tunnel: w459 -> [w464]
                  tunnel: w458 -> [w463]
                  tunnel: [w460] -> w457
                  tunnel: [w462] -> w456
                  tunnel: [w461] -> w455
                  tunnel: w457 -> [w475]
                  tunnel: w456 -> [w468]
                  tunnel: w455 -> [w469]
                  tunnel: w454 -> [w480]
                  tunnel: w453 -> [w479]
                  tunnel: [w466] -> w452
                  tunnel: [w470] -> w451
                  tunnel: [w469] -> w450
                  tunnel: w449 -> [w467]
                  tunnel: [w468] -> w447
                  tunnel: [w466] -> w445
                  tunnel: w444 -> [w465]
                  tunnel: [w465] -> w443
                  tunnel: w447 -> [w486]
                  tunnel: [w485] -> w446
                  tunnel: w445 -> [w484]
                  tunnel: w443 -> [w483]
                  frame #0 {
                    # "Get Final ACPR Value"
                    n87 = call "EXA_Get_ACPR.vi"("error in"=w464, "VISA resource name"=w463) -> ("error out"=w462:errorcluster, "ACP Sorted"=w460:dbl[], "VISA resource name"=w461:refnum<visa-resource-name>)  [unwired: 6 in, 1 out]
                  }
                  frame #1 {
                    # "Evaluate Results"
                    n88 = Index Array(array=w475, index=2) -> (element=w481:dbl)
                    n89 = Index Array(array=w475, index=1) -> (element=w474:dbl)
                    n90 = Index Array(array=w475, index=3) -> (element=w478:dbl)
                    n91 = Build Array (concatenate)(w467, w475) -> (w466:dbl[][])
                    "ACPR Data" <- w466
                    n92 = Greater Or Equal?(x=w481, y=w480) -> (x >= y?=w473:bool)
                    n93 = Less Or Equal?(x=w478, y=w479) -> (x <= y?=w471:bool)
                    n94 = Less Or Equal?(x=w474, y=w479) -> (x <= y?=w472:bool)
                    n95 = Compound Arithmetic op=AND(w473, w472, w471) -> (w470:bool)
                  }
                  frame #2 {
                    n96 = local read "Active ACPR Refnum"() -> (w487:refnum<vi>)
                    n97 = property class="Clust (strict)"(reference=w487, error in=w486) -> (reference out=w490:refnum<vi>, error out=w489:errorcluster, "Value"=w488:T12)
                    n98 = Bundle By Name(cluster=w488, "RFPAL PMU\nResults"=w483, "ACPR Data"=w484) -> (w491:T12)
                    n99 = property class="Clust (strict)"(reference=w490, error in=w489, "Value"=w491) -> (error out=w485:errorcluster)  [unwired: 1 out]
                  }
                }
              }
            }
          }
          "In Range?" <- w230
          "RF Frequency" <- w224
        }
      }
    }
    frame #2 {
      n100 = flat-sequence {
        tunnel: [w502] -> w499
        tunnel: [w501] -> w497
        tunnel: w498 -> [w501]
        tunnel: w492 -> [w500]
        tunnel: w499 -> [w508]
        tunnel: w497 -> [w507]
        tunnel: [w504] -> w494
        tunnel: [w505] -> w493
        tunnel: [w514] -> w496
        tunnel: w493 -> [w514]
        frame #0 {
          # "Disable Tx"
          n101 = call "TTA_MATLAB_RFIC_TX_Enable.vi"("Channels"=string[] [], "error in"=w500) -> ("error out"=w502:errorcluster)  [unwired: 12 in, 1 out]
        }
        frame #1 {
          # "Turn off MXG output"
          n102 = call "MXG_Set_RF_Output_State.vi"("error in"=w508, "RF Output State"="OFF", "VISA resource name"=w507) -> ("error out"=w504:errorcluster, "VISA resource name"=w505:refnum<visa-resource-name>)  [unwired: 7 in]
        }
        frame #2 {
          n103 = local read "RFPAL PMU\nResults"() -> (w511:dbl[])
          n104 = local read "RF Frequency"() -> (w512:dbl[])
          n105 = local read "ACPR Data"() -> (w513:dbl[][])
          n106 = local read "In Range?"() -> (w510:bool[])
          n107 = Bundle("ACPR Data"=w513, "RF Frequency"=w512, "RFPAL PMU\nResults"=w511, "In Range?"=w510) -> (→"ACPR\nResults":T1)  [unwired: 1 in]
        }
      }
    }
  }
  n108 = flat-sequence {
    tunnel: w15 -> [w517]
    tunnel: w14 -> [w516]
    tunnel: w7 -> [w515]
    frame #0 {
      "error out" <- w516
      "MXG VISA Resource Out" <- w515
      "EXA VISA Resource Out" <- w517
    }
  }
